vi "simx Set Object Int Parameter.vi"(6 "operationMode":i32, 7 "parameterValue":i32, 8 "error in (no error)":errorcluster, 9 "parameterID":i32, 10 "objectHandle":i32, 11 "clientID":i32) -> (0 "error out":errorcluster, 3 "function return":i32)   [LabVIEW 2019, in "PXL_V-REP.lvlib"]
doc: "EXTAPI_DLLEXPORT simxInt simxSetObjectIntParameter(simxInt clientID,simxInt objectHandle,simxInt parameterID,simxInt parameterValue,simxInt operationMode);"
uses:
  PXL_V-REP.lvlib
  <userlib>/V-REP/remoteApi.dll
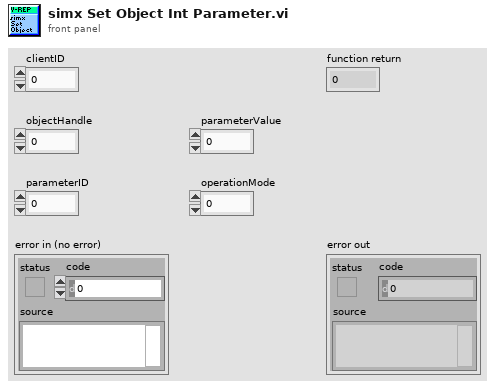
[diagram p1: front panel]
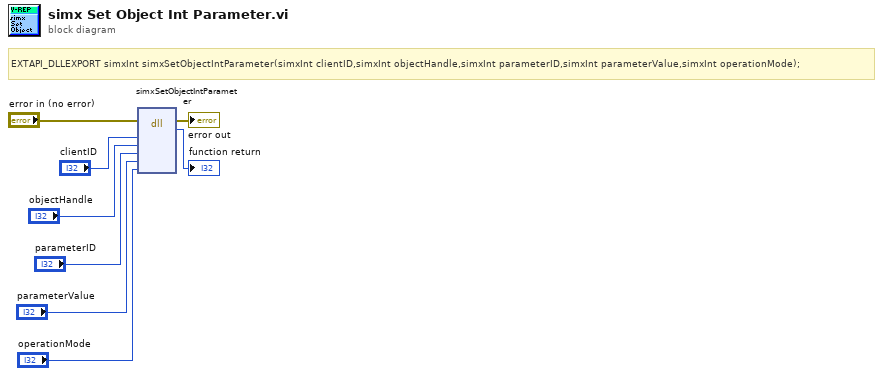
[diagram p0: block diagram]
diagram:
  # "EXTAPI_DLLEXPORT simxInt simxSetObjectIntParameter(simxInt clientID,simxInt objectHandle,simxInt parameterID,simxInt parameterValue,simxInt operationMode);"
  n1 = dll-call lib="C:/Program Files (x86)/National Instruments/LabVIEW 2019/user.lib/V-REP/remoteApi.*" fn="simxSetObjectIntParameter"(error in="error in (no error)", "clientID"="clientID", "objectHandle"="objectHandle", "parameterID"="parameterID", "parameterValue"="parameterValue", "operationMode"="operationMode") -> (error out=→"error out":errorcluster, →"function return":i32)  [unwired: 7 in, 1 out]
